vi "MAC DEF.vi"(0 "System no.":i32=1 min=1 max=4 step=1, 2 "Macro name":string, 5 "error in":errorcluster) -> (19 "error out":errorcluster)   [LabVIEW 2026]
doc: "Define autostart macro. To disable the autostart macro, \"Macro name\" must be an empty string.\n\nE-516: Autostart macro definition will not be saved to FLASH until WPA.vi was run. Changes not saved with WPA are only present in RAM and will be lost when the controller is powered off.\n\nE-816: Autostart macro definition will not be saved to FLASH until WPA.vi was run. Changes not saved with WPA are only present in RAM and will be lost when the controller is powered off. This command cannot be issued to a slave. Check controller manual to find out if MAC DEF is supported.\n\nC-887, F-206, M-8X0: Only for GCS syntax version = GCS 2.0 or higher (check with CSV?.vi. If CSV?.vi is not supported, syntax version is GCS 1.0)."
panel:
  # "Define autostart macro. To disable the autostart macro,\n\"Macro name\" must be an empty string."
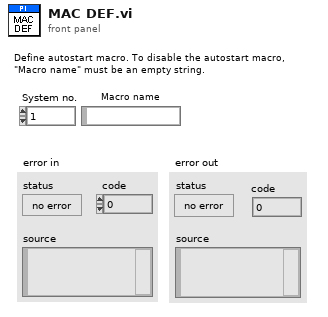
[diagram p1: front panel]
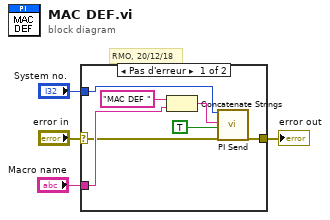
[diagram p0: block diagram]
diagram:
  # "RMO, 20/12/18"
  n1 = case shown="Pas d'erreur" "error in" {
    selector: "error in" -> [w5 w12]
    tunnel: "System no." -> [w11 _]
    tunnel: [w10 w12] -> w3
    tunnel: "Macro name" -> [w9 _]
    frame No Error {
      n2 = Concatenate Strings("MAC DEF ", w9) -> (w6:string)
      n3 = call "PI Send.vi"("System no."=w11, "String to send"=w6, "Attach termination char.?"=TRUE ("Attach Linefeed?"), "error in"=w5) -> ("error out"=w10:errorcluster)  [unwired: 2 in, 13 out]
    }
    frame Error {
    }
  }
  "error out" <- w3
